vi "myRIO_BRig_RT_dataMTrig_init.vi"() -> (2 "output_dataMTrig":u16[](array[numeric]))   [LabVIEW 2014]
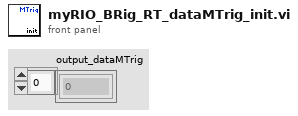
[diagram p1: front panel]
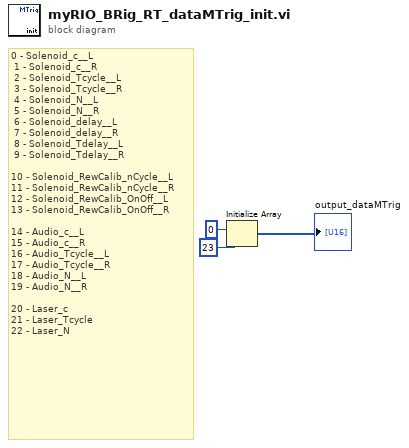
[diagram p0: block diagram]
diagram:
  # "0 - Solenoid_c__L\n 1 - Solenoid_c__R\n 2 - Solenoid_Tcycle__L\n 3 - Solenoid_Tcycle__R\n 4 - Solenoid_N__L\n 5 - Solenoid_N__R\n 6 - Solenoid_delay__L\n 7 - Solenoid_delay__R\n 8 - Solenoid_Tdelay__L\n 9 - Solenoid_Tdelay__R\n\n10 - Solenoid_RewCalib_nCycle__L\n11 - Solenoid_RewCalib_nCycle__R\n12 - Solenoid_RewCalib_OnOff__L\n13 - Solenoid_RewCalib_OnOff__R\n\n14 - Audio_c__L\n15 - Audio_c__R\n16 - Audio_Tcycle__L\n17 - Audio_Tcycle__R\n18 - Audio_N__L\n19 - Audio_N__R\n\n20 - Laser_c\n21 - Laser_Tcycle\n22 - Laser_N"
  n1 = Initialize Array(u16 0 ("element"), 23 ("dimension size")) -> (→"output_dataMTrig":u16[])
